vi "Teleop.vi"(8 "Error In":errorcluster) -> (0 "Error Out":errorcluster, 1 "Stop program and write to file":bool, 2 "SWITCH TO AUTONOMOUS 2":bool)   [LabVIEW 2013]
panel:
  in  "Teleop Comment":bool
  in  "Defense?":string(combo)="None"
  in  "Can they catch?":string(combo)="No"
  in  "SWITCH TO AUTONOMOUS":bool=TRUE
  in  "Stop Program and Write to File":bool
  in  "Can they pick up the ball?":string(combo)="No"
  in  "Missed Shots":dbl
  in  "Over Truss With Catch":dbl
  out "Assists":dbl
  in  "Over the Truss Pass":dbl
  out "Bottom Goal":dbl
  out "Top Goal":dbl
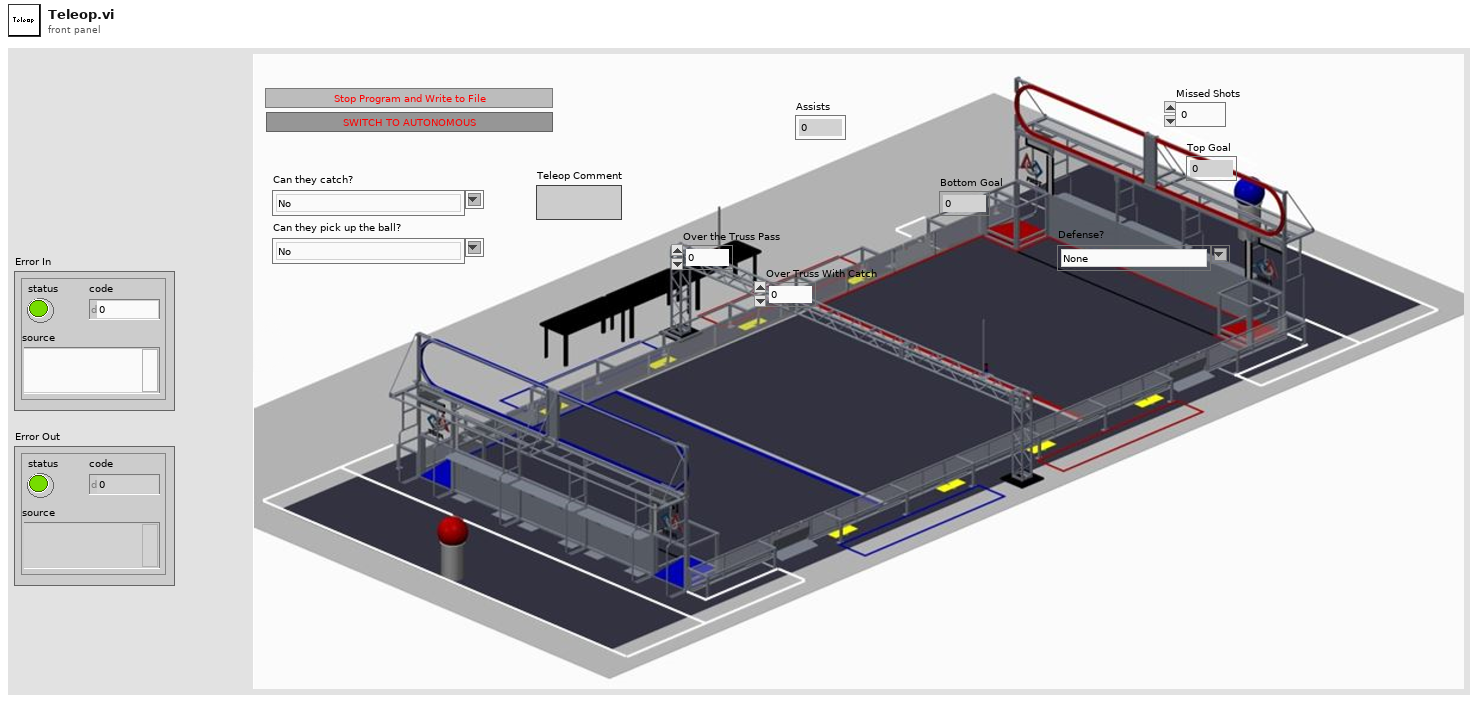
[diagram p1: front panel]
types:
  T1 = cluster{"Missed Shots":dbl, "Over Truss With Catch":dbl, "Over the Truss Pass":dbl, "Defense?":string, "Can they pick up the ball?":string, "Can they catch?":string}
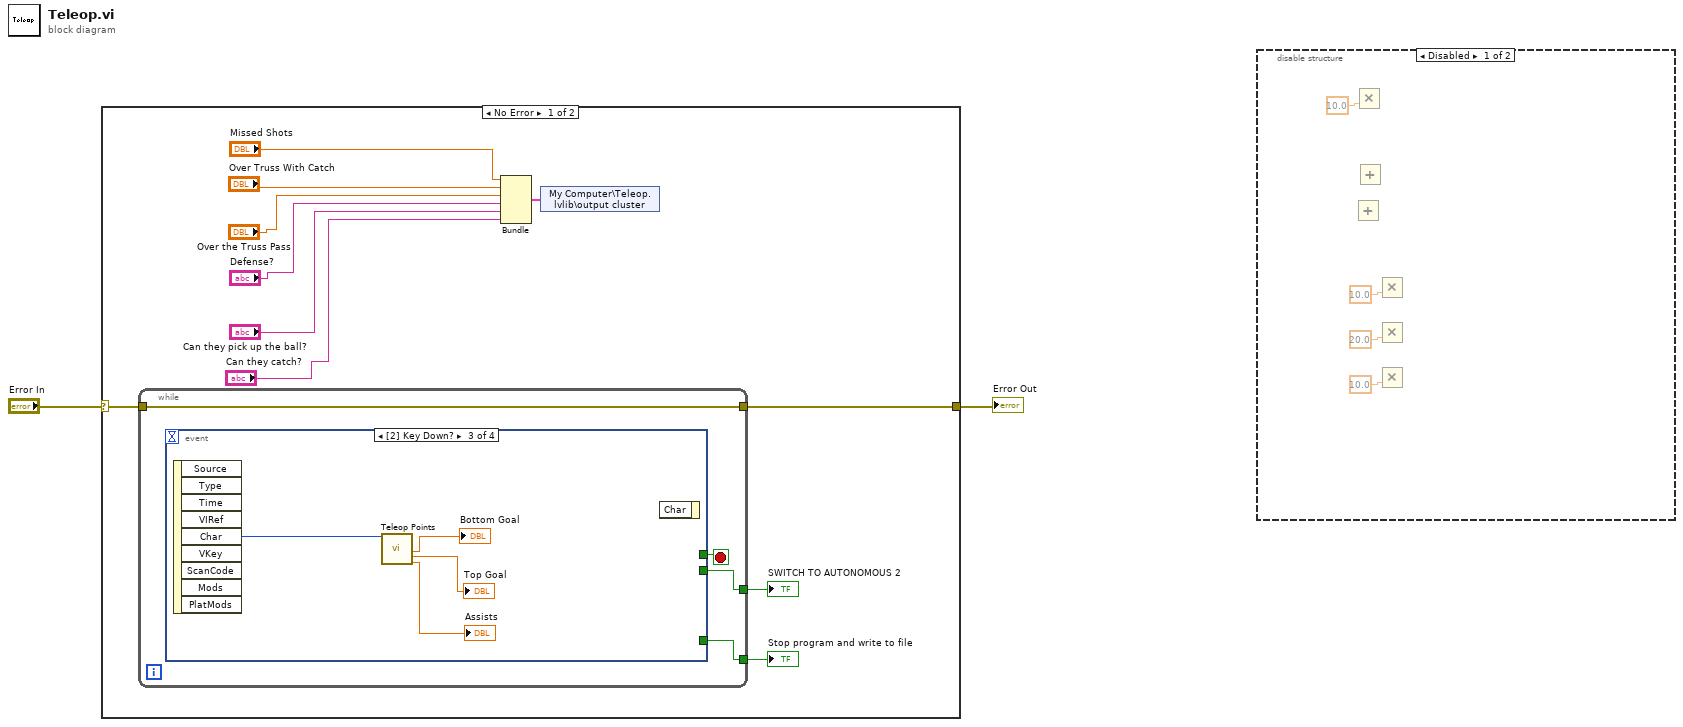
[diagram p0: block diagram]
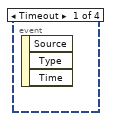
[diagram p2: hidden frame]
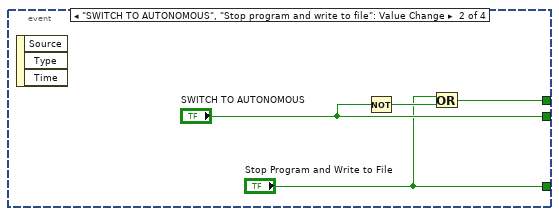
[diagram p3: hidden frame]
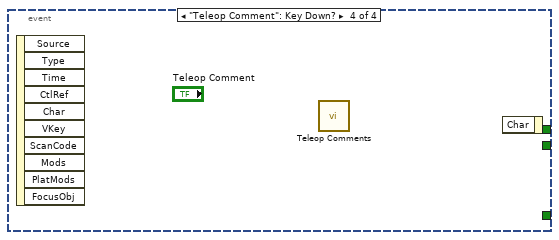
[diagram p4: hidden frame]
diagram:
  n1 = case shown="No Error" "Error In" {
    selector: "Error In" -> [w11 w26]
    tunnel: [w10 w26] -> w1
    frame No Error {
      n2 = while {
        tunnel: [w15] -> w13
        tunnel: [w14] -> w12
        tunnel: w11 -> [w17]
        tunnel: [w17] -> w10
        stop <- w16 stop-if-true
        n3 = event shown="[2] Key Down?" {
          selector: _ -> [_ _ _ _]
          dyn-events: _ -> [_ _ _ _]
          timeout: _ -> [_ _ _ _]
          tunnel: [_ w20 _ _] -> w16
          tunnel: [_ "SWITCH TO AUTONOMOUS" _ _] -> w15
          tunnel: [_ "Stop Program and Write to File" _ _] -> w14
          event Timeout {
            n4 = event-data() -> ()  [unwired: 1 in, 3 out]
          }
          event "SWITCH TO AUTONOMOUS", "Stop program and write to file": Value Change {
            n5 = event-data() -> ()  [unwired: 1 in, 3 out]
            n6 = Not(x="SWITCH TO AUTONOMOUS") -> (.not. x?=w21:bool)
            n7 = Or(x="Stop Program and Write to File", y=w21) -> (x .or. y?=w20:bool)
          }
          event Key Down? {
            n8 = event-data() -> ("Char"=w23:i16)  [unwired: 1 in, 8 out]
            n9 = call "Teleop Points.vi"("Char in"=w23) -> ("Bottom Goal"=→"Bottom Goal":dbl, "Top Goal"=→"Top Goal":dbl, "Assists"=→"Assists":dbl)  [unwired: 15 in, 1 out]
            n10 = event-data() -> ()  [unwired: 2 in, 1 out]
          }
          event "Teleop Comment": Key Down? {
            n11 = event-data() -> ()  [unwired: 1 in, 10 out]
            n12 = call "Teleop Comments.vi"() -> ()  [unwired: 11 in, 1 out]
            n13 = event-data() -> ()  [unwired: 2 in, 1 out]
          }
        }
      }
      "Stop program and write to file" <- w12
      "SWITCH TO AUTONOMOUS 2" <- w13
      n14 = Bundle("Missed Shots"="Missed Shots", "Over Truss With Catch"="Over Truss With Catch", "Over the Truss Pass"="Over the Truss Pass", "Defense?"="Defense?", "Can they pick up the ball?"="Can they pick up the ball?", "Can they catch?"="Can they catch?") -> (w3:T1)  [unwired: 1 in]
      n15 = shared-variable "My Computer\\Teleop.lvlib\\output cluster"(w3) -> ()  [unwired: 1 in, 1 out]
    }
    frame Error {
    }
  }
  "Error Out" <- w1
  n16 = disable-structure shown="Disabled" {
    frame Disabled {
      n17 = Add() -> ()  [unwired: 2 in, 1 out]
      n18 = Multiply(y=10.0) -> ()  [unwired: 1 in, 1 out]
      n19 = Add() -> ()  [unwired: 2 in, 1 out]
      n20 = Multiply(y=10.0) -> ()  [unwired: 1 in, 1 out]
      n21 = Multiply(y=20.0) -> ()  [unwired: 1 in, 1 out]
      n22 = Multiply(y=10.0) -> ()  [unwired: 1 in, 1 out]
    }
    frame Enabled {
    }
  }
